vi "OpenG Slice 1D Array Template.vi"(5 "slice":string caption="subset (i:j)", 6 "array":dbl[](array[numeric]) format="%.2f") -> (1 "subarray (array[i:j])":dbl[](array[numeric]) format="%.2f")   [LabVIEW 2012]
doc: "Returns a subset from <B>array</B>. <B>subset</B> has the following syntax:\n\narray[subset] = subarray\n\nsubset is a range and is of the form \"i:j\" where i and j are integers\nif i is ommitted it is assumed to be zero. If j is ommitted it is assumed to be length(array)\nif i or j are negative numbers they are assumed to be refferenced from the end of the string.\nexamples:\n\nif array = [7,6,5,4,3,2,1]\n\nstring[2:] = [5,4,3,2,1]\nstring[:3] = [7,6,5]\nstring[-1] = [1]\nstring[4] = [3]\nstring[-4:-2] = [4,3]"
panel:
  # "[OpenG VI Tags] ***Do Not Remove***\nSVN Revision = 990\nSVN Revision Date = 2009-07-18 07:14:13 -0700 (Sat, 18 Jul 2009)\nPackage = oglib_array-3.0.0-1\nDepends = oglib_string-2.6-1"
  # "Slice 1D Array.vi\n\nReturns a subset from array\n\nPlease visit http://www.OpenG.org to learn about the\nOpen Source LabVIEW software movement.\n\nNOTICE -- YOU MUST LEAVE THIS NOTICE IN PLACE.  PER THE TERMS OF THE LICENSE BELOW, YOU MAY SUBLICENSE THIS SOFTWARE \nIN ANY WAY THAT DOES NOT CONFLICT WITH THIS LICENSE.\n\n### BSD License (http://www.opensource.org/licenses/bsd-license.php) Begin ###\n \nCopyright (c) 2002, Jim Kring <jim@jimkring.com>\nCopyright (c) 2002, Cal-Bay Systems, Inc. <info@calbay.com>\n\nAll rights reserved.\n\nRedistribution and use in source and binary forms, with or without modification, are permitted provided that the following conditions are met:\n\n    * Redistributions of source code must retain the above copyright notice, this list of conditions and the following disclaimer.\n    * Redistributions in binary form must reproduce the above copyright notice, this list of conditions and the following disclaimer in the \n       documentation and/or other materials provided with the distribution.\n    * Neither the name of SciWare, James Kring, Inc., nor the names of its contributors may be used to endorse or promote products derived \n       from this software without specific prior written permission.\n\nTHIS SOFTWARE IS PROVIDED BY THE COPYRIGHT HOLDERS AND CONTRIBUTORS \"AS IS\" AND ANY EXPRESS OR IMPLIED WARRANTIES, \nINCLUDING, BUT NOT LIMITED TO, THE IMPLIED WARRANTIES OF MERCHANTABILITY AND FITNESS FOR A PARTICULAR PURPOSE ARE \nDISCLAIMED. IN NO EVENT SHALL THE COPYRIGHT OWNER OR CONTRIBUTORS BE LIABLE FOR ANY DIRECT, INDIRECT, INCIDENTAL,\n SPECIAL, EXEMPLARY, OR CONSEQUENTIAL DAMAGES (INCLUDING, BUT NOT LIMITED TO, PROCUREMENT OF SUBSTITUTE GOODS OR \nSERVICES; LOSS OF USE, DATA, OR PROFITS; OR BUSINESS INTERRUPTION) HOWEVER CAUSED AND ON ANY THEORY OF LIABILITY, \nWHETHER IN CONTRACT, STRICT LIABILITY, OR TORT (INCLUDING NEGLIGENCE OR OTHERWISE) ARISING IN ANY WAY OUT OF THE USE \nOF THIS SOFTWARE, EVEN IF ADVISED OF THE POSSIBILITY OF SUCH DAMAGE.\n\n### BSD License End ###"
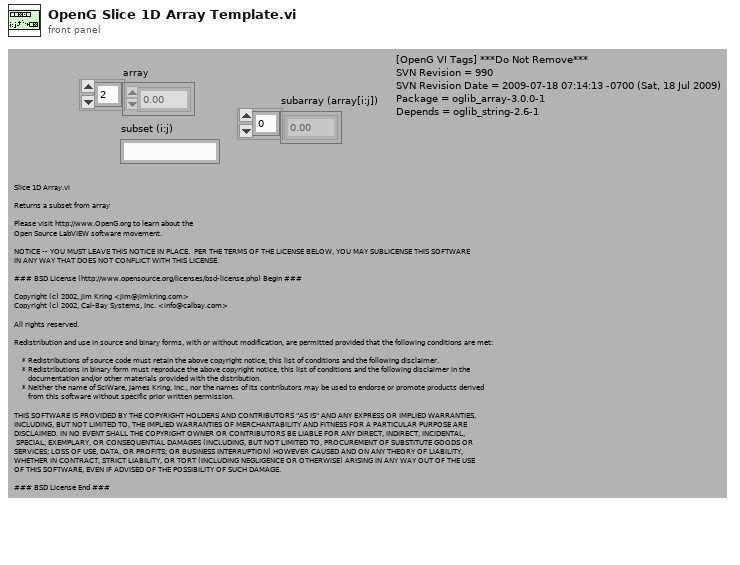
[diagram p1: front panel]
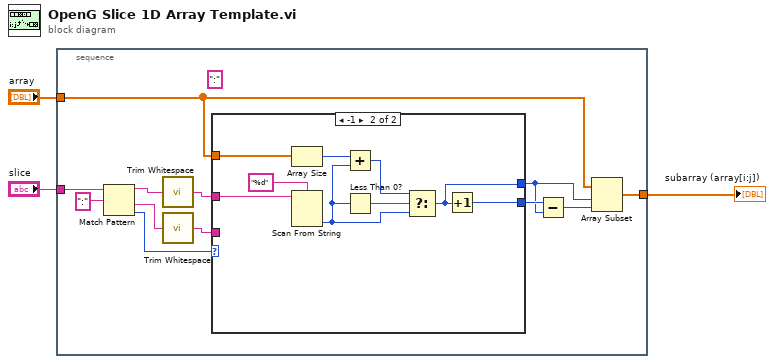
[diagram p0: block diagram]
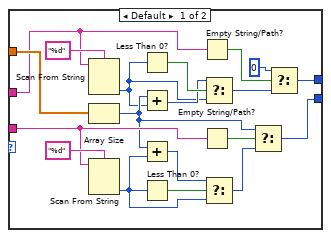
[diagram p2: hidden frame]
diagram:
  n1 = stacked-sequence {
    tunnel: [w13] -> w3
    tunnel: "array" -> [w12]
    tunnel: "slice" -> [w4]
    frame #0 {
      (unwired) ":"
      n2 = Match Pattern(string=w4, regular expression=":" ("search string/char (-)")) -> (before substring=w9:string, after substring=w7:string, offset past match=w10:i32)  [unwired: 2 out]
      n3 = call <vilib>:"Trim Whitespace.vi"("string"=w9) -> ("trimmed string"=w8:string)  [unwired: 1 in]
      n4 = call <vilib>:"Trim Whitespace.vi"("string"=w7) -> ("trimmed string"=w6:string)  [unwired: 1 in]
      n5 = case shown="-1" w10 {
        tunnel: [w25 w36] -> w15
        tunnel: [w26 w35] -> w14
        tunnel: w12 -> [w31 w41]
        tunnel: w8 -> [w28 w42]
        tunnel: w6 -> [w32 _]
        frame Default {
          n6 = Scan From String(format string="%d" ("Format String"), input string=w28) -> (output 1=w17:i32)  [unwired: 2 in, 4 out]
          n7 = Array Size(array=w31) -> (size(s)=w19:i32)
          n8 = Scan From String(format string="%d" ("Format String"), input string=w32) -> (output 1=w22:i32)  [unwired: 2 in, 4 out]
          n9 = Less Than 0?(x=w17) -> (x < 0?=w20:bool)
          n10 = Add(x=w19, y=w17) -> (x+y=w18:i32)
          n11 = Add(x=w19, y=w22) -> (x+y=w23:i32)
          n12 = Less Than 0?(x=w22) -> (x < 0?=w24:bool)
          n13 = Empty String/Path?(string/path=w28) -> (empty?=w30:bool)
          n14 = Empty String/Path?(string/path=w32) -> (empty?=w34:bool)
          n15 = Select(t=w18, s=w20, f=w17) -> (s? t:f=w16:i32)
          n16 = Select(t=w23, s=w24, f=w22) -> (s? t:f=w21:i32)
          n17 = Select(t=w19, s=w34, f=w21) -> (s? t:f=w25:i32)
          n18 = Select(t=0 ("length"), s=w30, f=w16) -> (s? t:f=w26:i32)
        }
        frame -1 {
          n19 = Array Size(array=w41) -> (size(s)=w39:i32)
          n20 = Scan From String(format string="%d" ("Format String"), input string=w42) -> (output 1=w37:i32)  [unwired: 2 in, 4 out]
          n21 = Add(x=w39, y=w37) -> (x+y=w38:i32)
          n22 = Less Than 0?(x=w37) -> (x < 0?=w40:bool)
          n23 = Select(t=w38, s=w40, f=w37) -> (s? t:f=w35:i32)
          n24 = Increment(x=w35) -> (x+1=w36:i32)
        }
      }
      n25 = Subtract(x=w15, y=w14) -> (x-y=w5:i32)
      n26 = Array Subset(array=w12, index=w14, length=w5) -> (w13:dbl[])
    }
  }
  "subarray (array[i:j])" <- w3
